vi "PLC_comm_test.vi"() -> ()   [LabVIEW 2018]
uses:
  <vilib>/OPCUA/controls/NodeId.ctl
  <vilib>/OPCUA/NI OPC UA Client.lvlib
panel:
  out "Retransmission count":i32
  out "Led OK comm":bool
  out "Relative Motor position Arduino":dbl
  out "Data Info":string
  out "PLC error out":errorcluster
  out "error out":errorcluster
  out "read buffer":string
  in  "VISA resource name":refnum<visa-resource-name>
  in  "baud rate (115200)":u32=115200
  in  "Direction":bool
  in  "Relative Motor position PLC":dbl
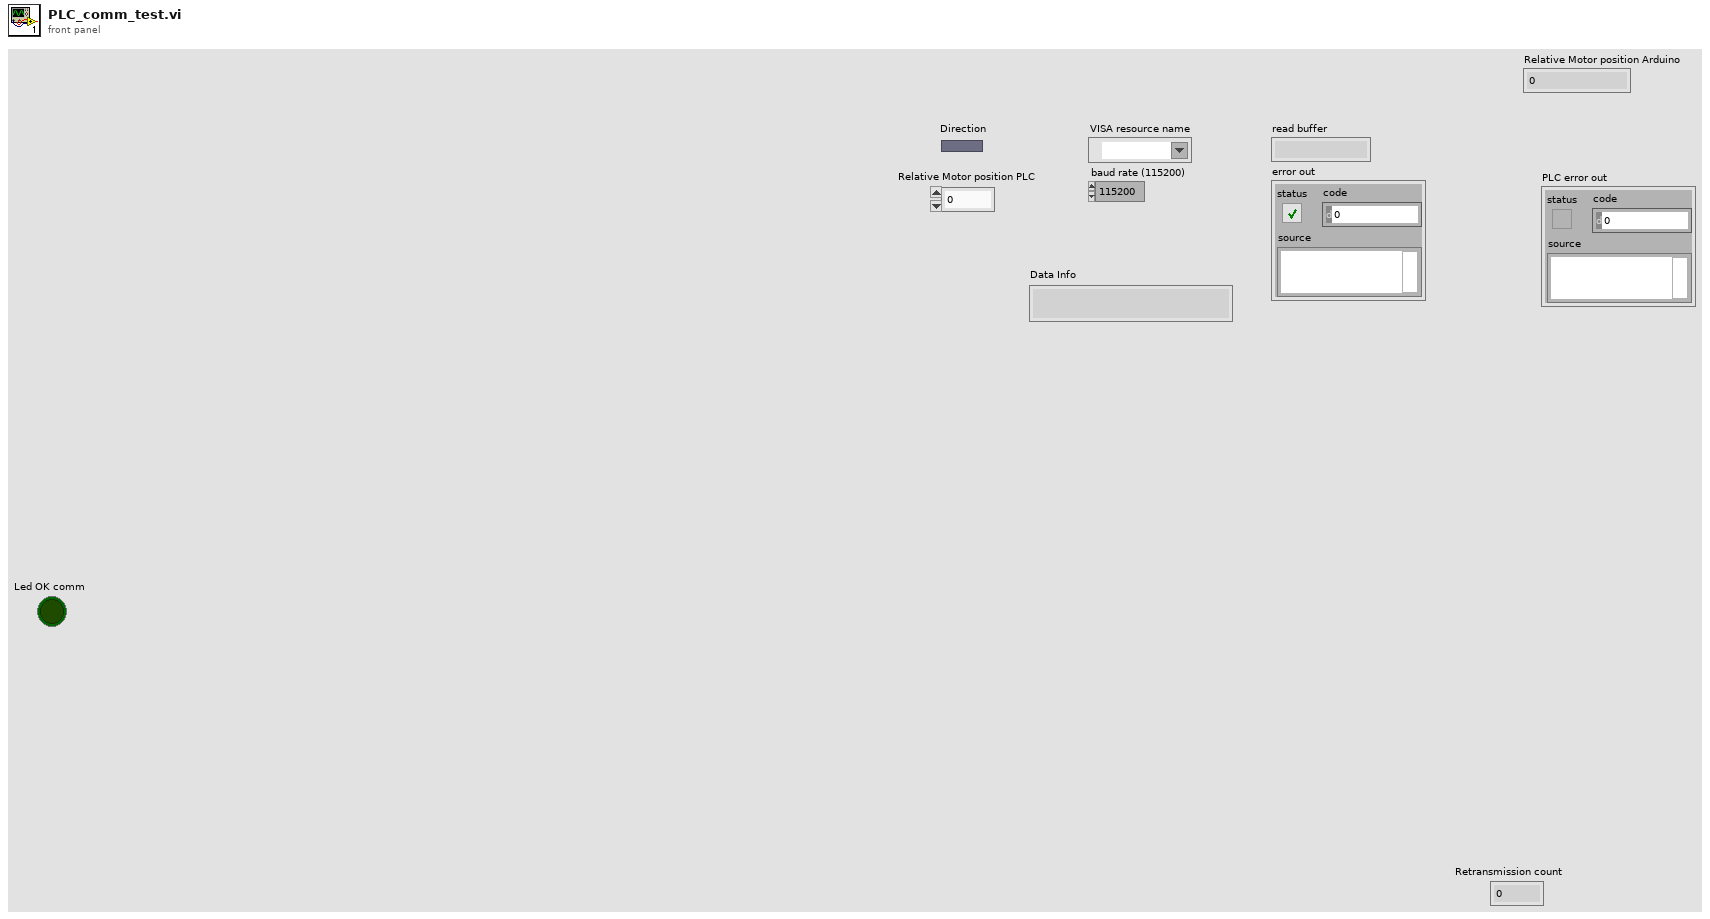
[diagram p1: front panel]
types:
  T1 = cluster{"message mode":enum16{"None", "Sign", "Sign and Encrypt"}, "security":enum16{"Basic256", "Basic128Rsa15"}}
  T2 = typedef "OPC UA Client Refnum.ctl" = refnum<k21>
  T3 = typedef "NodeId.ctl" = string
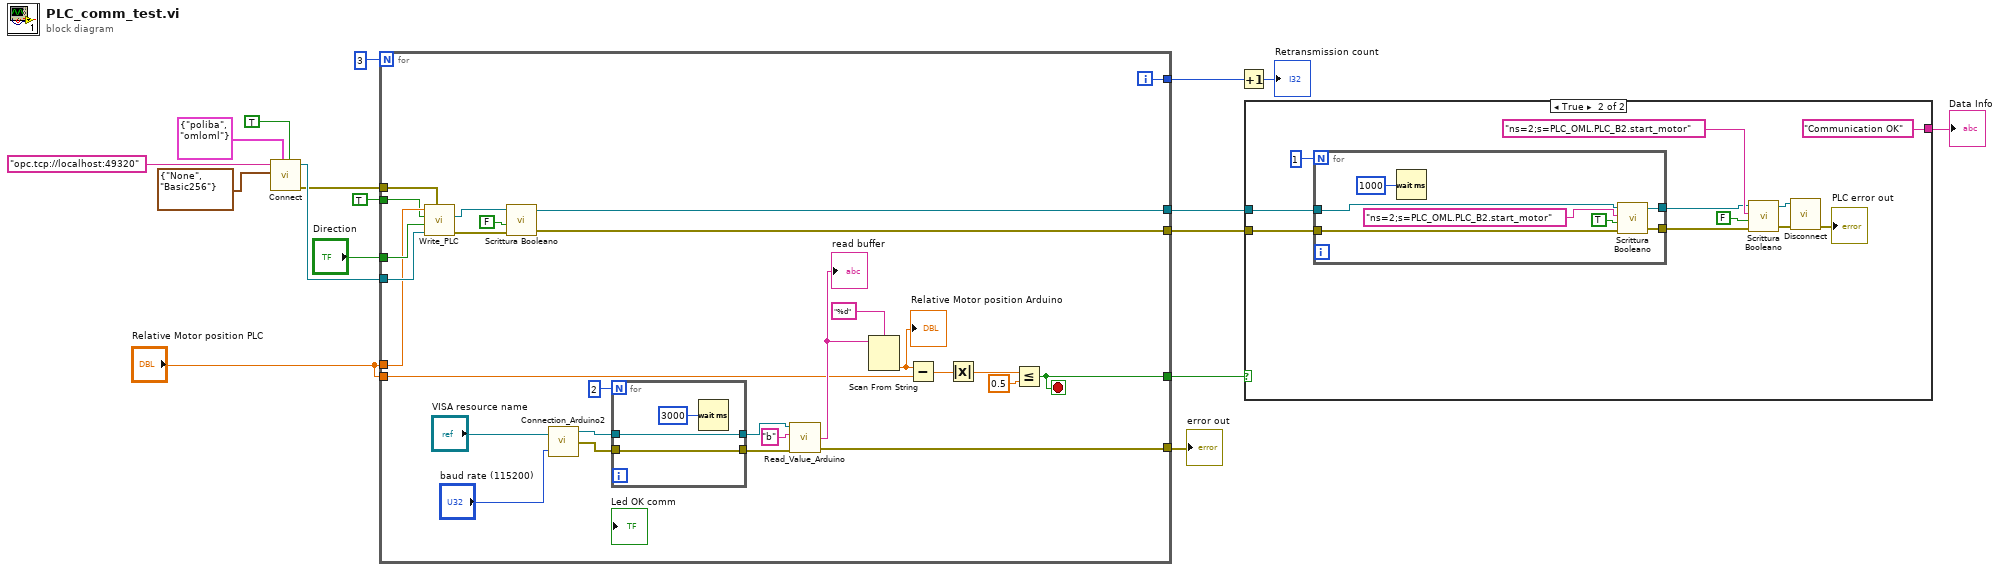
[diagram p0: block diagram]
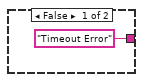
[diagram p2: hidden frame]
diagram:
  n1 = call <vilib>:"Connect.vi"("trust any server (F)"=TRUE, "username/password"=cluster{"username":string, "password":string} {"username"="poliba", "password"="omloml"}, "security policy"=T1 {"message mode"=enum."None", "security"=enum."Basic256"}, "server endpoint URL"="opc.tcp://localhost:49320") -> ("error out"=w6:errorcluster, "OPC UA client refnum out"=w9:T2)  [unwired: 5 in, 1 out]
  n2 = for {
    N: 3 -> [_]
    tunnel: [w45] -> w10
    tunnel: w9 -> [w28]
    tunnel: "Direction" -> [w27]
    tunnel: "Relative Motor position PLC" -> [w26]
    tunnel: TRUE ("Start_communication") -> [w25]
    tunnel: w6 -> [w24]
    tunnel: [w23] -> w5
    tunnel: "Relative Motor position PLC" -> [w22]
    tunnel: [w21] -> w3
    tunnel: [w20] -> w2
    tunnel: [w19] -> w1
    i -> [w45]
    stop <- w19 stop-if-true
    n3 = call "Write_PLC.vi"("error in"=w24, "OPC UA client refnum out"=w28, "Direction"=w27, "Start_communication"=w25, "Relative_Motor_position"=w26) -> ("error out"=w37:errorcluster, "OPC UA client refnum out 2"=w38:T2)  [unwired: 2 out]
    n4 = call "Scrittura Booleano.vi"("OPC UA client refnum in"=w38, "Value"=FALSE, "error in (no error)"=w37) -> ("OPC UA client refnum out"=w21:T2, "error out"=w20:errorcluster)  [unwired: 2 in, 1 out]
    n5 = call "Connection_Arduino2.vi"("VISA resource name"="VISA resource name", "baud rate (9600)"="baud rate (115200)") -> ("VISA resource name out"=w39:refnum<visa-resource-name>, "error out"=w40:errorcluster)  [unwired: 1 out]
    n6 = for {
      N: 2 -> [_]
      tunnel: w39 -> [w47]
      tunnel: [w47] -> w42
      tunnel: [w46] -> w41
      tunnel: w40 -> [w46]
      n7 = Wait (ms)(milliseconds to wait=u32 3000) -> ()  [unwired: 1 out]
    }
    n8 = call "Read_Value_Arduino.vi"("VISA resource name"=w42, "write buffer"="b", "error in (no error)"=w41) -> ("concatenated string"=w44:string, "error out"=w23:errorcluster)  [unwired: 1 in, 2 out]
    "read buffer" <- w44
    n9 = Scan From String(format string="%d", input string=w44) -> (output 1=w33:dbl)  [unwired: 3 in, 3 out]
    "Relative Motor position Arduino" <- w33
    n10 = Subtract(x=w33, y=w22) -> (x-y=w34:dbl)
    n11 = Absolute Value(x=w34) -> (abs(x)=w35:dbl)
    n12 = Less Or Equal?(x=w35, y=0.5) -> (x <= y?=w19:bool)
  }
  "error out" <- w5
  n13 = Increment(x=w10) -> (x+1=→"Retransmission count":i32)
  n14 = case shown="True" w1 {
    tunnel: ["Timeout Error" ("Data Info") "Communication OK" ("Data Info 2")] -> w13
    tunnel: w3 -> [_ w51]
    tunnel: w2 -> [_ w50]
    frame False {
    }
    frame True {
      n15 = for {
        N: 1 -> [_]
        tunnel: [w64] -> w54
        tunnel: [w63] -> w53
        tunnel: w51 -> [w62]
        tunnel: w50 -> [w61]
        n16 = Wait (ms)(milliseconds to wait=u32 1000) -> ()  [unwired: 1 out]
        n17 = call "Scrittura Booleano.vi"("OPC UA client refnum in"=w62, "node ID"=T3 "ns=2;s=PLC_OML.PLC_B2.start_motor", "Value"=TRUE, "error in (no error)"=w61) -> ("OPC UA client refnum out"=w64:T2, "error out"=w63:errorcluster)  [unwired: 1 in, 1 out]
      }
      n18 = call "Scrittura Booleano.vi"("OPC UA client refnum in"=w54, "node ID"=T3 "ns=2;s=PLC_OML.PLC_B2.start_motor", "Value"=FALSE, "error in (no error)"=w53) -> ("OPC UA client refnum out"=w58:T2, "error out"=w57:errorcluster)  [unwired: 1 in, 1 out]
      n19 = call <vilib>:"Disconnect.vi"("error in (no error)"=w57, "OPC UA client refnum in"=w58) -> ("error out"=→"PLC error out":errorcluster)  [unwired: 9 in]
    }
  }
  "Data Info" <- w13
